vi "CH_LM Test.vi"() -> ()   [LabVIEW 2012, in "CH_LM.lvlib"]
doc: "You can use this VI as starting point for your own application.\n\n<B>Hint:</B> This VI will startand stop the CH_LM ActiveX Control.vi automatially."
uses:
  CH_LM.lvlib
  CH_LM/CH_LM Communication Mode.ctl
  CH_LM/CH_LM BaudRates.ctl
  CH_LM/CH_LM Parity.ctl
  CH_LM/CH_LM SerialConfiguration.ctl
panel:
  in  "Serial Configuration\n(19200,N,8,1)":T1={"Baud Rate"=19200, "Parity"=0, "Data Bits"=8, "Stop Bits"=1} {"Parity" items=["None", "Odd", "Even"]; "Baud Rate" items=["9600"=9600, "19200"=19200, "38400"=38400, "57600"=57600, "115200"=115200]}
  in  "GPIB Board (0)":i16
  in  "Communication Mode":T4
  in  "Intervall / ms":i32
  out "Lock timed out?":bool
  out "stopped":bool
  out "last update":timestamp
  out "loop":i32
  in  "Reset":bool
  out "error out":errorcluster
  in  "stop":bool
  in  "Address":i32=1
  in  "Serial Number":string
  in  "Reset? (F: No)":bool
  in  "ID Query? (T: Yes)":bool
  in  "update":bool
  in  "set":bool
  in  "Wavelength Correction (disable)":bool
  in  "Wavelength / nm":u32
  out "Wavelength / nm":u32
  out "Wavelength Correction":bool
  in  "Option (Value)":enum16{"MINIMUM", "Value", "MAXIMUM"}(ring)=enum."Value"
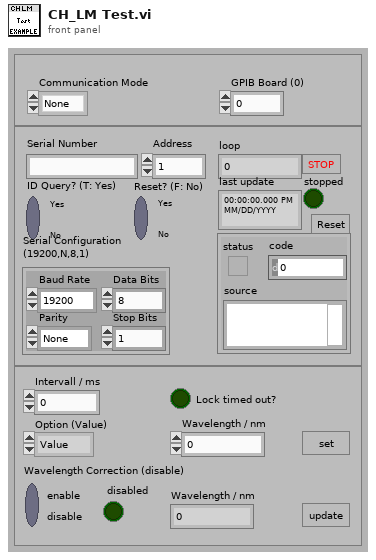
[diagram p1: front panel]
types:
  T1 = typedef "CH_LM.lvlib/CH_LM SerialConfiguration.ctl" = cluster{"Baud Rate":T2, "Parity":T3, "Data Bits":u16, "Stop Bits":u16}
  T2 = typedef "CH_LM.lvlib/CH_LM BaudRates.ctl" = u32
  T3 = typedef "CH_LM.lvlib/CH_LM Parity.ctl" = u16
  T4 = typedef "CH_LM.lvlib/CH_LM Communication Mode.ctl" = enum16{"None", "USB", "GPIB", "RS232"}
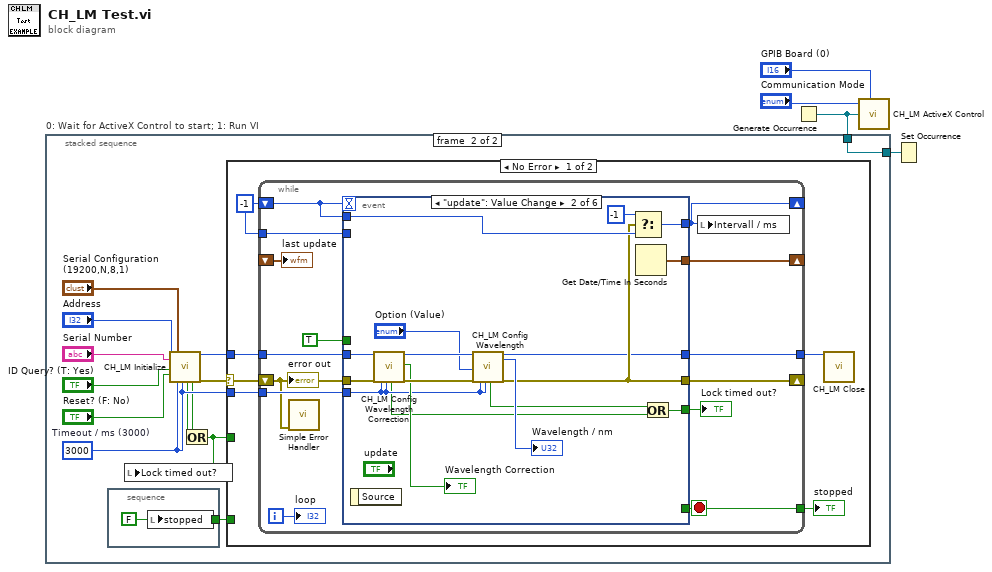
[diagram p0: block diagram]
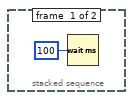
[diagram p2: hidden frame]
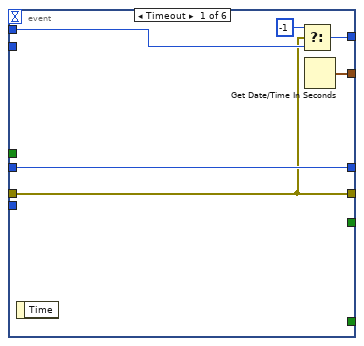
[diagram p3: hidden frame]
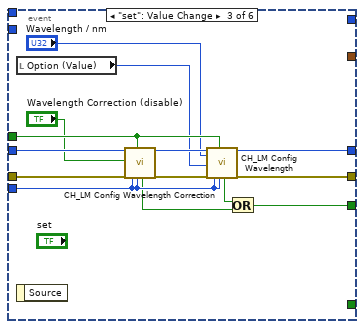
[diagram p4: hidden frame]
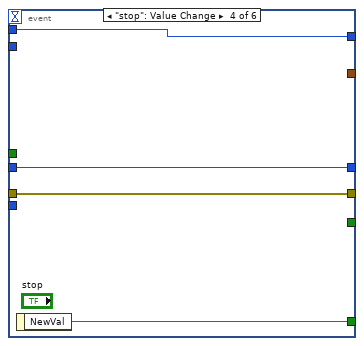
[diagram p5: hidden frame]
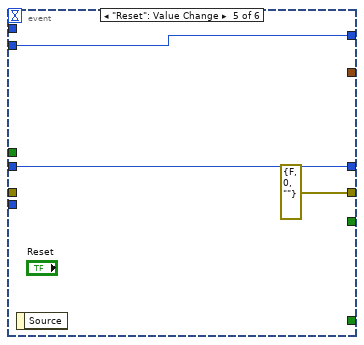
[diagram p6: hidden frame]
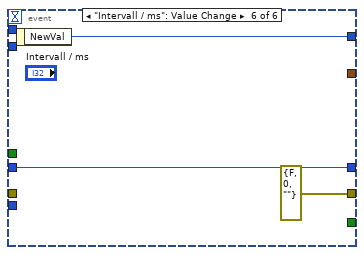
[diagram p7: hidden frame]
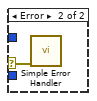
[diagram p8: hidden frame]
diagram:
  n1 = Generate Occurrence() -> (w2:refnum<k4>)
  n2 = stacked-sequence "0: Wait for ActiveX Control to start; 1: Run VI" {
    tunnel: [_ w7] -> w1
    tunnel: w2 -> [_ w7]
    frame #0 {
      n3 = Wait (ms)(milliseconds to wait=u32 100) -> ()  [unwired: 1 out]
    }
    frame #1 {
      w14 = 3000  # Timeout / ms (3000)
      n4 = stacked-sequence {
        tunnel: [w19] -> w11
        frame #0 {
          w19 = FALSE ("stopped")
          n5 = local write "stopped"(w19) -> ()
        }
      }
      n6 = call "CH_LM Initialize.vi"("Address"="Address", "Serial Number"="Serial Number", "ID Query (True)"="ID Query? (T: Yes)", "Reset (False)"="Reset? (F: No)", "Serial Configuration\n(19200,N,8,1)"="Serial Configuration\n(19200,N,8,1)", "Timeout / ms (3000)"=w14, "Lock Timeout / ms (1000)"=w14) -> ("Lock timed out"=w13:bool, "timed out?"=w12:bool, "Meter Index"=w16:i32, "error out"=w15:errorcluster)  [unwired: 1 in, 8 out]
      n7 = Or(x=w12, y=w13) -> (x .or. y?=w8:bool)
      n8 = local write "Lock timed out?"(w8) -> ()
      n9 = case shown="No Error" w15 {
        selector: w15 -> [w21 w87]
        tunnel: w16 -> [w22 _]
        tunnel: w14 -> [w20 _]
        tunnel: w8 -> [_ _]
        tunnel: w11 -> [_ _]
        frame No Error {
          w23 = -1
          n10 = while {
            tunnel: w22 -> [w39]
            tunnel: [w38] -> w25
            shift-right: [w37] -> _
            shift-left: w21 -> [w31]
            tunnel: w20 -> [w36]
            tunnel: [w34] -> w24
            shift-right: [w26] -> _
            shift-left: w23 -> [w33]
            tunnel: w23 -> [w32]
            shift-right: [w30] -> _
            shift-left: _ -> [w29]
            i -> [w35]
            stop <- w34 stop-if-true
            n11 = call <vilib>:"Simple Error Handler.vi"("error in (no error)"=w31) -> ()  [unwired: 1 in, 8 out]
            n12 = event shown="[1] \"update\": Value Change" {
              selector: _ -> [_ _ _ _ _ _]
              dyn-events: _ -> [_ _ _ _ _ _]
              timeout: w33 -> [_ _ _ _ _ _]
              tunnel: [_ _ _ w80 _ _] -> w34
              tunnel: w39 -> [w41 w53 w76 w79 w82 w85]
              tunnel: w31 -> [w40 w52 w73 w78 _ _]
              tunnel: [w41 w49 w74 w79 w82 w85] -> w38
              tunnel: [w40 w50 w66 w78 errorcluster {"status"=FALSE, "code"=0, "source"=""} ("error out") errorcluster {"status"=FALSE, "code"=0, "source"=""} ("error out")] -> w37
              tunnel: w36 -> [_ w51 w71 _ _ _]
              tunnel: [w45 w62 _ w77 w81 w84] -> w26
              tunnel: w33 -> [w44 w61 _ w77 _ _]
              tunnel: w32 -> [_ _ _ _ w81 _]
              tunnel: [w42 w59 _ _ _ _] -> w30
              tunnel: TRUE ("Action (query)") -> [_ _ w70 _ _ _]
              tunnel: [_ w48 w63 _ _ _] -> w27
              event Timeout {
                n13 = event-data() -> ()  [unwired: 2 out]
                n14 = Select(t=-1, s=w40, f=w44) -> (s? t:f=w45:i32)
                n15 = Get Date/Time In Seconds() -> (seconds since 1Jan1904=w42:timestamp)
              }
              event "update": Value Change {
                n16 = event-data() -> ()  [unwired: 2 out]
                n17 = call "CH_LM Config Wavelength Correction.vi"("Meter Index"=w53, "error in (no error)"=w52, "Timeout / ms (3000)"=w51, "Lock Timeout / ms (1000)"=w51) -> ("Lock timed out"=w46:bool, "Meter Index"=w57:i32, "Wavelength Correction"=→"Wavelength Correction":bool, "error out"=w58:errorcluster)  [unwired: 2 in, 10 out]
                n18 = call "CH_LM Config Wavelength.vi"("Meter Index"=w57, "Option (Value)"="Option (Value)", "error in (no error)"=w58, "Timeout / ms (3000)"=w51, "Lock Timeout / ms (1000)"=w51) -> ("Lock timed out"=w47:bool, "Meter Index"=w49:i32, "Wavelength / nm"=→"Wavelength / nm":u32, "error out"=w50:errorcluster)  [unwired: 2 in, 9 out]
                n19 = Select(t=-1, s=w50, f=w61) -> (s? t:f=w62:i32)
                n20 = Get Date/Time In Seconds() -> (seconds since 1Jan1904=w59:timestamp)
                n21 = Or(x=w47, y=w46) -> (x .or. y?=w48:bool)
              }
              event "set": Value Change {
                n22 = local read "Option (Value)"() -> (w67:enum16{"MINIMUM", "Value", "MAXIMUM"})
                n23 = event-data() -> ()  [unwired: 2 out]
                n24 = call "CH_LM Config Wavelength Correction.vi"("Meter Index"=w76, "Wavelength Correction (disable)"="Wavelength Correction (disable)", "error in (no error)"=w73, "Timeout / ms (3000)"=w71, "Action (query)"=w70, "Lock Timeout / ms (1000)"=w71) -> ("Lock timed out"=w64:bool, "Meter Index"=w75:i32, "error out"=w72:errorcluster)  [unwired: 11 out]
                n25 = call "CH_LM Config Wavelength.vi"("Meter Index"=w75, "Wavelength / nm"="Wavelength / nm", "Option (Value)"=w67, "error in (no error)"=w72, "Timeout / ms (3000)"=w71, "Action (query)"=w70, "Lock Timeout / ms (1000)"=w71) -> ("Lock timed out"=w65:bool, "Meter Index"=w74:i32, "error out"=w66:errorcluster)  [unwired: 10 out]
                n26 = Or(x=w65, y=w64) -> (x .or. y?=w63:bool)
              }
              event "stop": Value Change {
                n27 = event-data() -> ("NewVal"=w80:bool)  [unwired: 1 out]
              }
              event "Reset": Value Change {
                n28 = event-data() -> ()  [unwired: 2 out]
              }
              event "Intervall / ms": Value Change {
                n29 = event-data() -> ("NewVal"=w84:i32)  [unwired: 1 out]
              }
            }
            "Lock timed out?" <- w27
            n30 = local write "Intervall / ms"(w26) -> ()
            "error out" <- w31
            "loop" <- w35
            "last update" <- w29
          }
          "stopped" <- w24
          n31 = call "CH_LM Close.vi"("Meter Index"=w25) -> ()  [unwired: 1 in, 18 out]
        }
        frame Error {
          n32 = call <vilib>:"Simple Error Handler.vi"("error in (no error)"=w87) -> ()  [unwired: 1 in, 8 out]
        }
      }
    }
  }
  n33 = call "CH_LM ActiveX Control.vi"("Communication Mode"="Communication Mode", "GPIB Board (0)"="GPIB Board (0)", "MonitorStop Occurrence"=w2) -> ()  [unwired: 1 in, 2 out]
  n34 = Set Occurrence(w1) -> ()
